vi "LMTD.vi"(1 "Air Down/In Temp":dbl[unit], 2 "Air  UP/Out Temp":dbl[unit], 3 "Water Down/out Temp":dbl[unit], 4 "Water Up/In Temp":dbl[unit]) -> (0 "LMTD":dbl[unit])   [LabVIEW 2018]
panel:
  out "AIR temp Evaporator In":dbl[unit]
  out "AIR temp Evaporator Out":dbl[unit]
  out "LMTD":dbl[unit](knob) scale=0.0..5.0
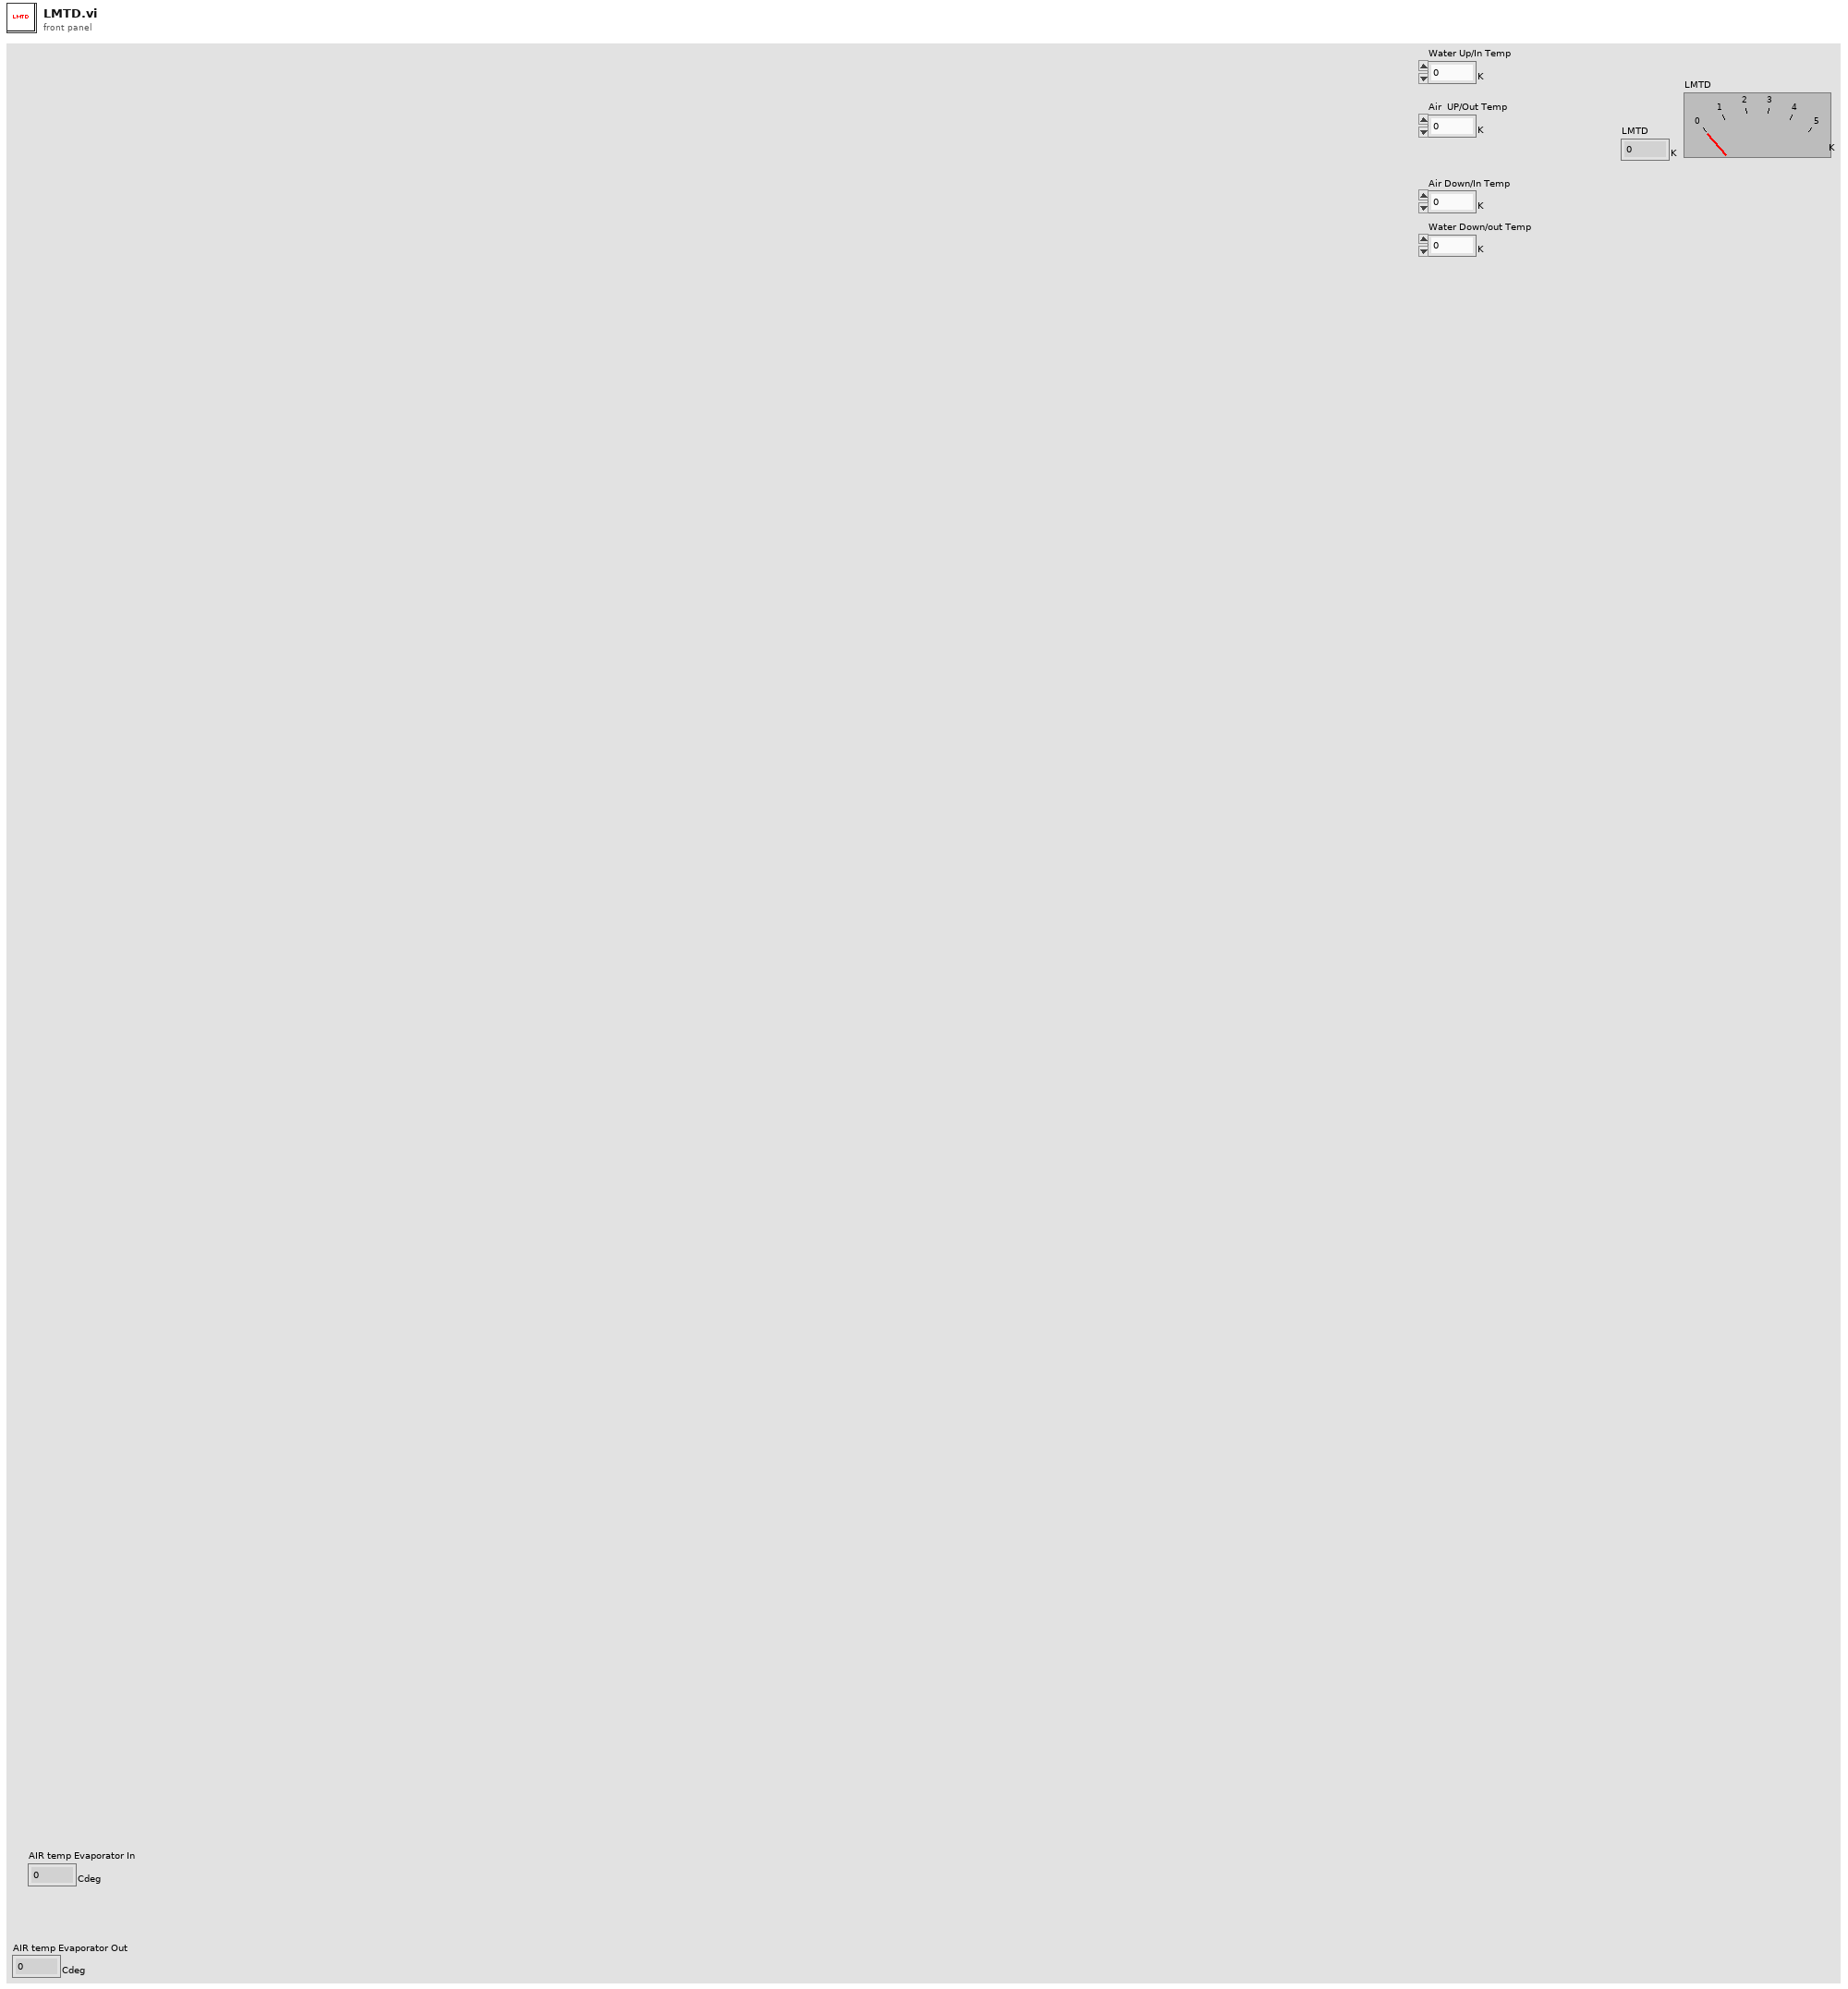
[diagram p1: front panel]
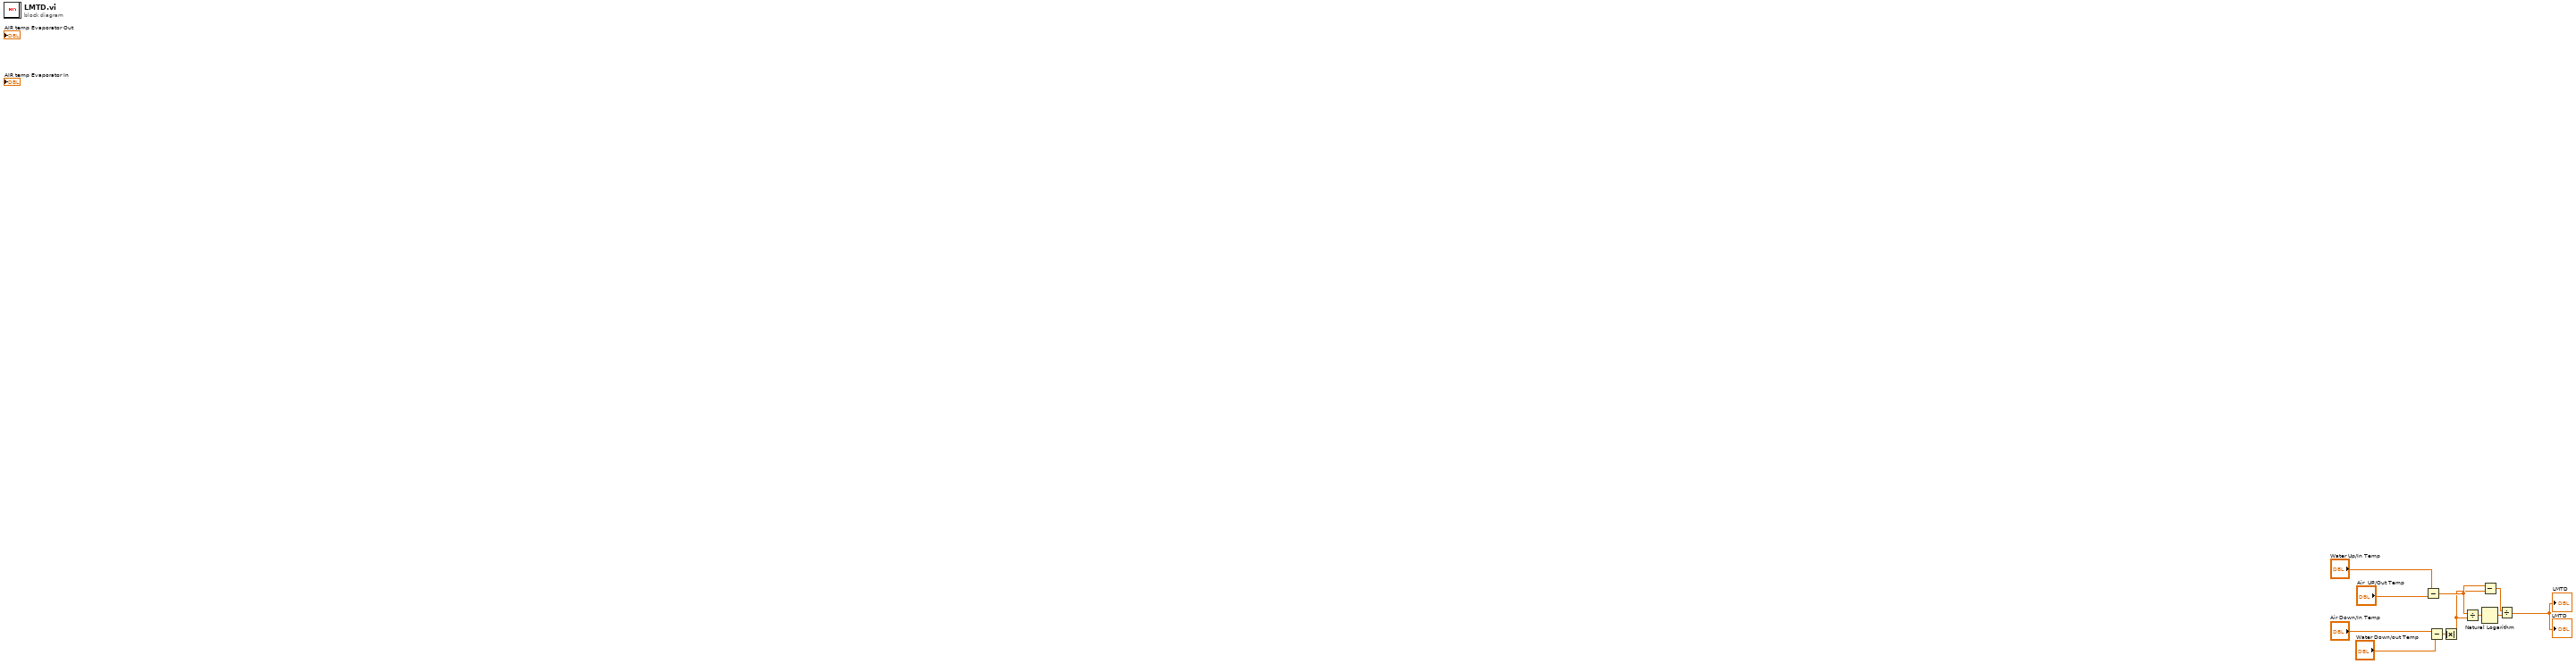
[diagram p0: block diagram]
diagram:
  n1 = Subtract(x="Water Up/In Temp", y="Air  UP/Out Temp") -> (x-y=w9:dbl[unit])
  n2 = Subtract(x="Air Down/In Temp", y="Water Down/out Temp") -> (x-y=w8:dbl[unit])
  n3 = Absolute Value(x=w8) -> (abs(x)=w7:dbl[unit])
  n4 = Divide(x=w9, y=w7) -> (x/y=w6:dbl)
  n5 = Natural Logarithm(1:w6) -> (0:w10:dbl)
  n6 = Subtract(x=w9, y=w7) -> (x-y=w11:dbl[unit])
  n7 = Divide(x=w11, y=w10) -> (x/y=→"LMTD" →"LMTD":dbl[unit])
